vi "Exp_ICCD_GetGateMode.vi"(8 "error in (no error)":errorcluster, 11 "LightField Automation in":refnum<class "LightField Automation.lvclass">) -> (0 "error out":errorcluster, 2 "Gate Mode":string, 3 "LightField Automation out":refnum<class "LightField Automation.lvclass">)   [LabVIEW 2013, in "LightField Automation.lvclass"]
uses:
  LightField Automation.lvclass
  C:/Program Files/Princeton Instruments/LightField/PrincetonInstruments.LightFieldAddInSupportServices.dll
  Program Files/Princeton Instruments/LightField/PrincetonInstruments.LightFieldAddInSupportServices.dll
  LightField Automation.lvclass/LightField Automation.ctl
  C:/Program Files/Princeton Instruments/LightField/AddInViews/PrincetonInstruments.LightFieldViewV3.dll
  Program Files/Princeton Instruments/LightField/AddInViews/PrincetonInstruments.LightFieldViewV3.dll
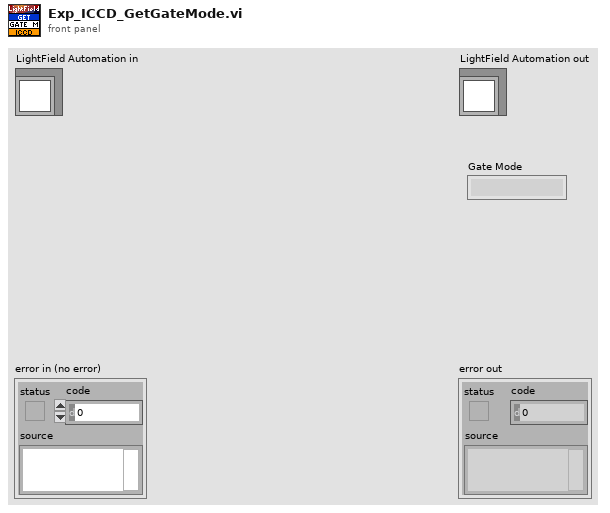
[diagram p1: front panel]
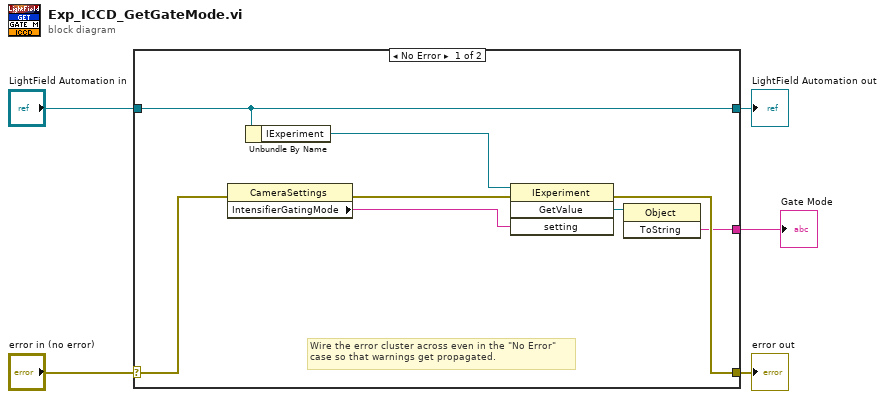
[diagram p0: block diagram]
diagram:
  n1 = case shown="No Error" "error in (no error)" {
    selector: "error in (no error)" -> [w10 w15]
    tunnel: [w11 w15] -> w4
    tunnel: [w13 w14] -> w2
    tunnel: "LightField Automation in" -> [w13 w14]
    tunnel: [w6 _] -> w1
    frame No Error {
      # "Wire the error cluster across even in the \"No Error\"\ncase so that warnings get propagated."
      n2 = property class="CameraSettings"(error in=w10) -> (error out=w9:errorcluster, "IntensifierGatingMode"=w8:string)  [unwired: 1 in, 1 out]
      n3 = Unbundle By Name(w13) -> ("IExperiment"=w12:refnum<k24>)
      n4 = invoke class="IExperiment" method="GetValue"(reference=w12, error in=w9, "setting"=w8) -> (error out=w11:errorcluster, "GetValue"=w7:refnum<k24>)  [unwired: 1 in, 2 out]
      n5 = invoke class="Object" method="ToString"(reference=w7) -> ("ToString"=w6:string)  [unwired: 2 in, 2 out]
    }
    frame Error {
    }
  }
  "error out" <- w4
  "LightField Automation out" <- w2
  "Gate Mode" <- w1
